vi "cam0-合并择优槽点组-2.vi"(9 "槽点组优先":T2(array[cluster]), 10 "槽点组初步":T2(array[cluster]), 11 "ImageIn":T1) -> (2 "槽点组合并":T2(array[cluster]), 3 "ImageOut":T1)   [LabVIEW 2018]
uses:
  <vilib>/vision/Image Controls.llb/IMAQ Image.ctl
panel:
  in  "显示槽点组":bool
  in  "同槽槽点最大距离":sgl=30.0
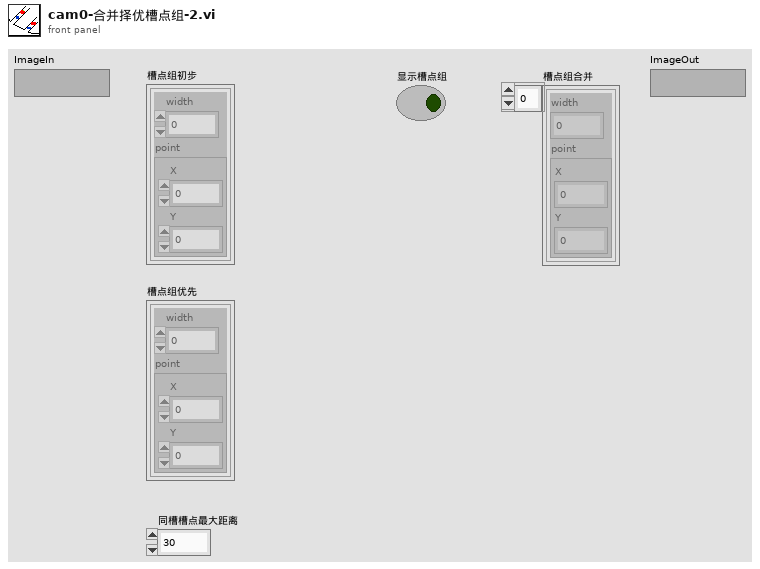
[diagram p1: front panel]
types:
  T1 = typedef "IMAQ Image.ctl" = refnum<image>
  T2 = cluster{"width":sgl, "point":cluster{"X":sgl, "Y":sgl}}[]
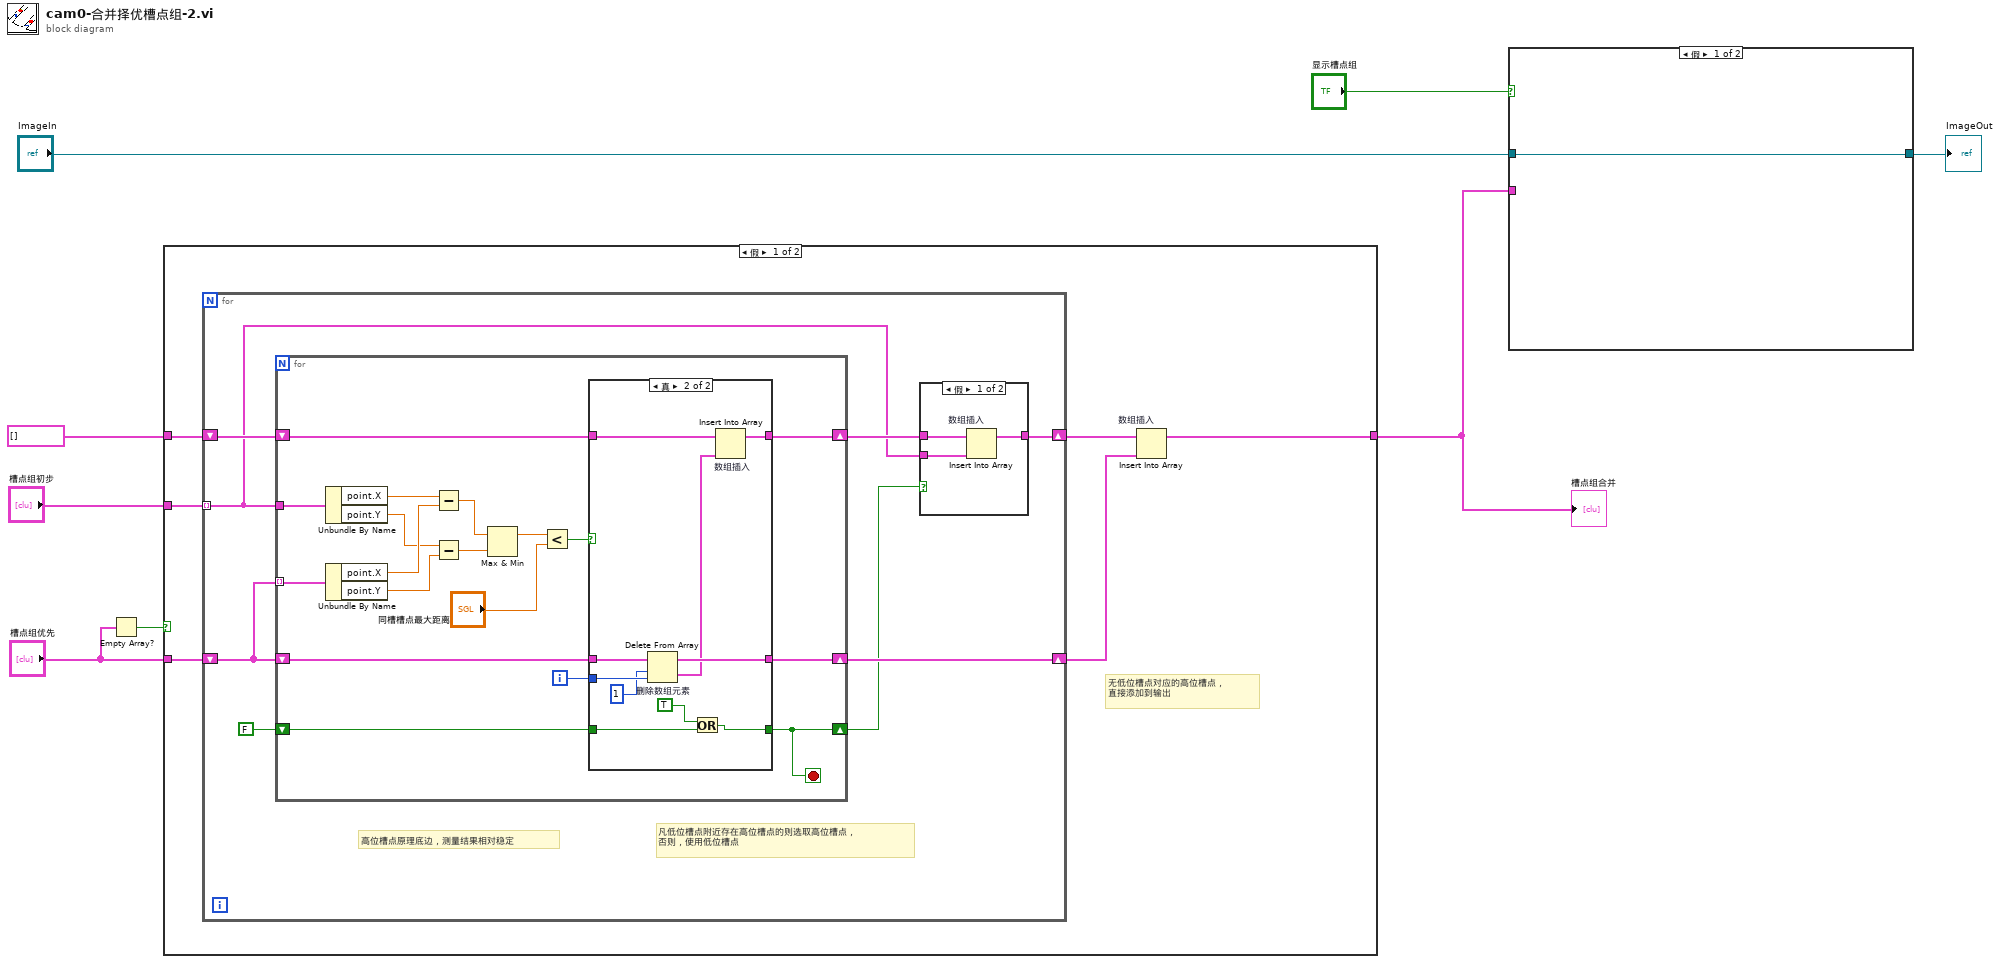
[diagram p0: block diagram]
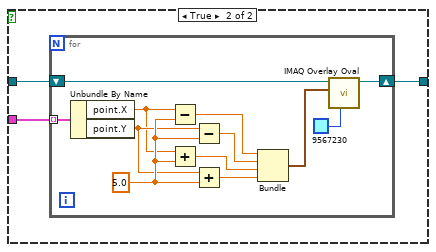
[diagram p2: hidden frame]
diagram:
  n1 = Empty Array?(array="槽点组优先") -> (empty?=w6:bool)
  n2 = case shown="假" w6 {
    tunnel: T2 [] ("槽点组1") -> [w14 _]
    tunnel: [w10 w58] -> w4
    tunnel: "槽点组优先" -> [w13 _]
    tunnel: "槽点组初步" -> [w12 w58]
    frame False {
      # "无低位槽点对应的高位槽点，\n直接添加到输出"
      n3 = for {
        tunnel: w12 -> [w15] mode=indexing
        shift-right: [w16] -> w11
        shift-left: w14 -> [w22]
        shift-right: [w21] -> w9
        shift-left: w13 -> [w20]
        # "高位槽点原理底边，测量结果相对稳定"
        # "凡低位槽点附近存在高位槽点的则选取高位槽点，\n否则，使用低位槽点"
        n4 = for {
          tunnel: w15 -> [w44]
          tunnel: w20 -> [w32] mode=indexing
          shift-right: [w34] -> w17
          shift-left: w22 -> [w35]
          shift-right: [w30] -> w21
          shift-left: w20 -> [w31]
          shift-right: [w27] -> w18
          shift-left: FALSE -> [w28]
          i -> [w29]
          stop <- w27 stop-if-true
          n5 = Unbundle By Name(w44) -> ("point.X"=w43:sgl, "point.Y"=w41:sgl)
          n6 = Unbundle By Name(w32) -> ("point.X"=w42:sgl, "point.Y"=w40:sgl)
          n7 = Subtract(x=w43, y=w42) -> (x-y=w39:sgl)
          n8 = Subtract(x=w41, y=w40) -> (x-y=w38:sgl)
          n9 = Max & Min(x=w39, y=w38) -> (max(x,y)=w37:sgl)  [unwired: 1 out]
          n10 = Less?(x=w37, y="同槽槽点最大距离") -> (x < y?=w33:bool)
          n11 = case shown="真" w33 {
            tunnel: w35 -> [w47 w57]
            tunnel: [w47 w56] -> w34
            tunnel: w31 -> [w46 w55]
            tunnel: [w46 w54] -> w30
            tunnel: w29 -> [_ w53]
            tunnel: w28 -> [w45 w50]
            tunnel: [w45 w48] -> w27
            frame False {
            }
            frame True {
              n12 = Delete From Array "删除数组元素"(array=w55, length=1 ("长度"), index=w53) -> (deleted portion=w51:T2, array with subset deleted=w54:T2)
              n13 = Or(x=TRUE, y=w50) -> (x .or. y?=w48:bool)
              n14 = Insert Into Array "数组插入"(array=w57, new element=w51) -> (w56:T2)  [unwired: 1 in]
            }
          }
        }
        n15 = case shown="假" w18 {
          tunnel: w17 -> [w25 w26]
          tunnel: [w24 w26] -> w16
          tunnel: w15 -> [w23 _]
          frame False {
            n16 = Insert Into Array "数组插入"(array=w25, new element=w23) -> (w24:T2)  [unwired: 1 in]
          }
          frame True {
          }
        }
      }
      n17 = Insert Into Array "数组插入"(array=w11, new element=w9) -> (w10:T2)  [unwired: 1 in]
    }
    frame True {
    }
  }
  "槽点组合并" <- w4
  n18 = case shown="假" "显示槽点组" {
    tunnel: w4 -> [_ w62]
    tunnel: "ImageIn" -> [w59 w61]
    tunnel: [w59 w60] -> w2
    frame False {
    }
    frame True {
      n19 = for {
        tunnel: w62 -> [w67] mode=indexing
        shift-right: [w63] -> w60
        shift-left: w61 -> [w64]
        w73 = sgl 5.0 ("y")
        n20 = Unbundle By Name(w67) -> ("point.X"=w70:sgl, "point.Y"=w72:sgl)
        n21 = Subtract(x=w70, y=w73) -> (x-y=w68:sgl)
        n22 = Add(x=w70, y=w73) -> (x+y=w71:sgl)
        n23 = Subtract(x=w72, y=w73) -> (x-y=w69:sgl)
        n24 = Add(x=w72, y=w73) -> (x+y=w74:sgl)
        n25 = Bundle(w68, w69, w71, w74) -> (w65:cluster{sgl, sgl, sgl, sgl})  [unwired: 1 in]
        n26 = call "IMAQ Overlay Oval"("Color"=u32 9567230, "Bounding Rectangle"=w65, "Image"=w64) -> ("Image Out"=w63:T1)  [unwired: 7 in, 1 out]
      }
    }
  }
  "ImageOut" <- w2
